vi "DSF.Shared.Configuration.Initialize.vi"(8 "error in (no error)":errorcluster, 9 "settings":T1, 10 "name":string, 11 "Configuration in":refnum<class "DSF.Shared.Configuration.lvclass">) -> (0 "error out":errorcluster, 3 "Configuration out":refnum<class "DSF.Shared.Configuration.lvclass">)   [LabVIEW 2017, in "DSF.Engine.lvlib" / "DSF.Shared.Configuration.lvclass"]
uses:
  DSF.Shared.Configuration.lvclass
  DSF Configuration API/1.0.0/Public/Controls/DSF Settings Info.ctl
  DSF.Shared.Configuration.lvclass/DSF.Shared.Configuration.ctl
  DSF Configuration API/1.0.0/DSF Configuration API.lvlib
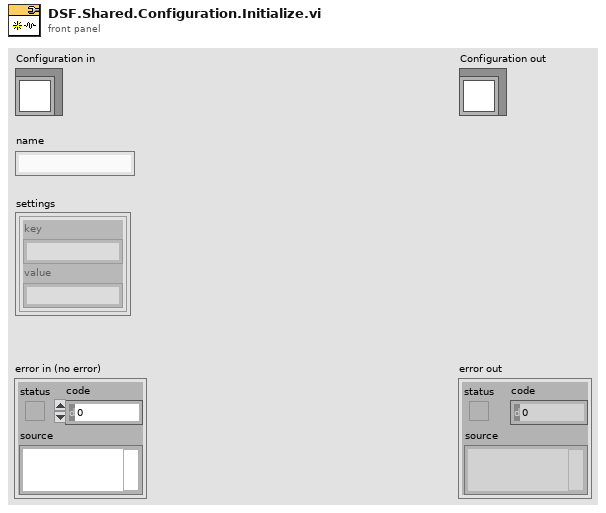
[diagram p1: front panel]
types:
  T1 = typedef "DSF Configuration API.lvlib/DSF Settings Info.ctl" = cluster{"key":string, "value":string}[]
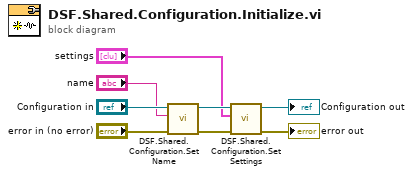
[diagram p0: block diagram]
diagram:
  n1 = call "DSF.Shared.Configuration.Set Name.vi"("name"="name", "Configuration in"="Configuration in") -> ("Configuration out"=w5:refnum<class "DSF.Shared.Configuration.lvclass">)  [unwired: 9 in]
  n2 = call "DSF.Shared.Configuration.Set Settings.vi"("settings"="settings", "Configuration in"=w5) -> ("Configuration out"=→"Configuration out":refnum<class "DSF.Shared.Configuration.lvclass">)  [unwired: 9 in]
  "error out" <- "error in (no error)"
